vi "Convolution OLD.vi"(0 "reference in":refnum<class "SigMath.lvclass">, 5 "error in (no error)":errorcluster) -> (14 "reference out":refnum<class "SigMath.lvclass">, 19 "error out":errorcluster)   [LabVIEW 2020, in "SigMath.lvclass"]
uses:
  SigMath.lvclass
  <vilib>/Analysis/2dsp.llb/1D Convolution (DBL).vi
  <vilib>/Analysis/NI_AALPro.lvlib
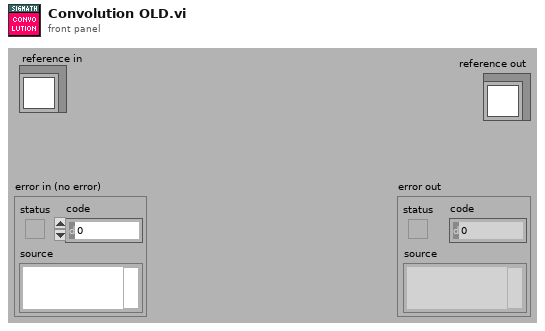
[diagram p1: front panel]
types:
  T1 = typedef "SigMath.lvclass/ObjectAttributesRef.ctl" = refnum<data-value>
  T2 = typedef "SigMath.lvclass/ObjectAttributes.ctl" = cluster{"SigMath Data":T3, "User CTRL Refs":T4}
  T3 = typedef "SigMath.lvclass/SigMath Data.ctl" = cluster{"New Time Data Obj?":bool, "GSwFormDSP":refnum<class "GSwFormDSP.lvclass">}
  T4 = typedef "SigMath.lvclass/SigMath User CTRL Refs.ctl" = cluster{"wForms":refnum<vi>, "Results wForms":refnum<vi>}
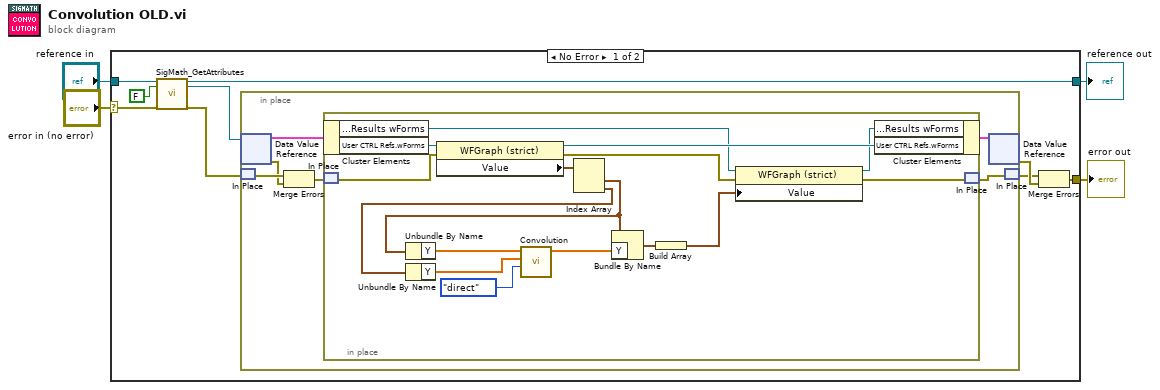
[diagram p0: block diagram]
diagram:
  n1 = case shown="No Error" "error in (no error)" {
    selector: "error in (no error)" -> [w9 w37]
    tunnel: [w13 w37] -> w3
    tunnel: [w8 w36] -> w1
    tunnel: "reference in" -> [w11 w36]
    frame No Error {
      n2 = call "SigMath_GetAttributes.vi"("reference in"=w11, "return data? (T)"=FALSE, "error in (no error)"=w9) -> ("reference out"=w8:refnum<class "SigMath.lvclass">, "attributes ref"=w7:T1, "error out"=w6:errorcluster)  [unwired: 13 in, 1 out]
      n3 = in-place {
        n4 = in-place-dvr #1(w7) -> (w18:T2, w16:errorcluster)
        n5 = in-place-match #2(w6) -> (w17:errorcluster)
        n6 = Merge Errors(w17, w16) -> (w15:errorcluster)
        n7 = in-place {
          n8 = in-place-cluster #3(w18) -> ("User CTRL Refs.Results wForms"=w31:refnum<vi>, "User CTRL Refs.wForms"=w34:refnum<vi>)
          n9 = in-place-match #4(w15) -> (w35:errorcluster)
          n10 = property class="WFGraph (strict)"(reference=w34, error in=w35) -> (reference out=w32:refnum<vi>, error out=w29:errorcluster, "Value"=w33:waveform(dbl)[])
          n11 = Index Array(array=w33) -> (element #1=w26:waveform(dbl), element #2=w28:waveform(dbl))  [unwired: 2 in]
          n12 = Unbundle By Name(w26) -> ("Y"=w27:dbl[])
          n13 = Unbundle By Name(w28) -> ("Y"=w20:dbl[])
          n14 = call-poly <vilib>:"Convolution.vi"("algorithm"=enum32{"direct", "frequency domain"}."direct", "Y"=w20, "X"=w27) -> ("X * Y"=w25:dbl[])  [unwired: 7 in, 1 out]
          n15 = Bundle By Name(cluster=w26, "Y"=w25) -> (w24:waveform(dbl))
          n16 = Build Array(w24) -> (w23:waveform(dbl)[])
          n17 = property class="WFGraph (strict)"(reference=w31, error in=w29, "Value"=w23) -> (reference out=w30:refnum<vi>, error out=w22:errorcluster)
          n18 = in-place-cluster #3("User CTRL Refs.Results wForms"=w30, "User CTRL Refs.wForms"=w32) -> (w19:T2)
          n19 = in-place-match #4(w22) -> (w14:errorcluster)
        }
        n20 = in-place-dvr #1(w19) -> (w12:errorcluster)  [unwired: 1 out]
        n21 = in-place-match #2(w14) -> (w5:errorcluster)
      }
      n22 = Merge Errors(w5, w12) -> (w13:errorcluster)
    }
    frame Error {
    }
  }
  "error out" <- w3
  "reference out" <- w1
